vi "Format table.vi"(11 "Table输入":refnum<vi>) -> ()   [LabVIEW 2016]
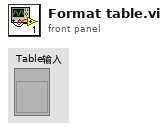
[diagram p1: front panel]
types:
  T1 = cluster{"Font Name:":string, "Size":i16, "Strikeout?":bool, "Italic?":bool, "Underline?":bool, "Outline?":bool, "Shadow?":bool, "Bold?":bool}
  T2 = enum16{"User-specified Font", "Application Font", "System Font", "Dialog Font"}
  T3 = typedef "LVFontTypeDef.ctl" = cluster{"Font Name":string, "Size":u16, "Bold":bool, "Italic":bool, "Underline":bool, "Strikeout":bool, "Color":u32}
  T4 = cluster{"left":i16, "top":i16, "right":i16, "bottom":i16}
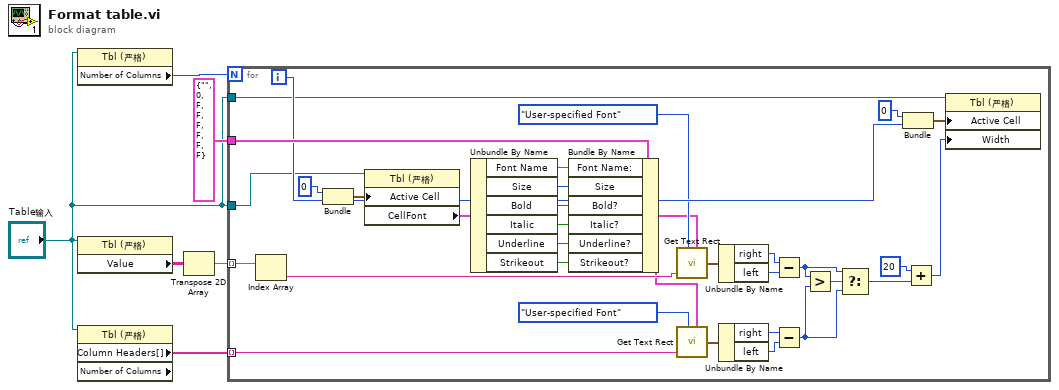
[diagram p0: block diagram]
diagram:
  n1 = property on="属性节点" class="Tbl (严格)"(reference="Table输入") -> ("Number of Columns"=w5:u32)  [unwired: 1 in, 2 out]
  n2 = property class="Tbl (严格)"(reference="Table输入") -> ("Value"=w6:string[][])  [unwired: 1 in, 2 out]
  n3 = property class="Tbl (严格)" props=["Column Headers[]", "Number of Columns"](reference="Table输入") -> ("Column Headers[]"=w1:string[])  [unwired: 1 in, 3 out]
  n4 = Transpose 2D Array(2D array=w6) -> (transposed array=w4:string[][])
  n5 = for {
    N: w5 -> [_]
    tunnel: w4 -> [w19] mode=indexing
    tunnel: T1 {"Font Name:"="", "Size"=0, "Strikeout?"=FALSE, "Italic?"=FALSE, "Underline?"=FALSE, "Outline?"=FALSE, "Shadow?"=FALSE, "Bold?"=FALSE} ("[user-specified font]") -> [w39]
    tunnel: "Table输入" -> [w33]
    tunnel: "Table输入" -> [w32]
    tunnel: w1 -> [w14] mode=indexing
    i -> [w38]
    n6 = Index Array(array=w19) -> (element=w18:string)  [unwired: 1 in]
    n7 = Bundle(0, w38) -> (w20:cluster{i32, i32})  [unwired: 1 in]
    n8 = property on="属性节点" class="Tbl (严格)"(reference=w33, "Active Cell"=w20) -> ("CellFont"=w21:T3)  [unwired: 1 in, 2 out]
    n9 = Unbundle By Name(w21) -> ("Font Name"=w31:string, "Size"=w30:u16, "Bold"=w29:bool, "Italic"=w28:bool, "Underline"=w27:bool, "Strikeout"=w26:bool)
    n10 = Bundle By Name(cluster=w39, "Font Name:"=w31, "Size"=w30, "Bold?"=w29, "Italic?"=w28, "Underline?"=w27, "Strikeout?"=w26) -> (w16:T1)
    n11 = call <vilib>:"Get Text Rect.vi"("desired font(Application)"=T2."User-specified Font", "text"=w18, "[user-specified font]"=w16) -> ("rect"=w24:T4)  [unwired: 6 in]
    n12 = call <vilib>:"Get Text Rect.vi"("desired font(Application)"=T2."User-specified Font", "text"=w14, "[user-specified font]"=w16) -> ("rect"=w11:T4)  [unwired: 6 in]
    n13 = Unbundle By Name(w24) -> ("right"=w23:i16, "left"=w22:i16)
    n14 = Unbundle By Name(w11) -> ("right"=w12:i16, "left"=w13:i16)
    n15 = Subtract(x=w23, y=w22) -> (x-y=w9:i16)
    n16 = Subtract(x=w12, y=w13) -> (x-y=w8:i16)
    n17 = Greater?(x=w9, y=w8) -> (0:w10:bool)
    n18 = Select(t=w9, s=w10, f=w8) -> (s? t:f=w7:i16)
    n19 = Bundle(0, w38) -> (w34:cluster{i32, i32})  [unwired: 1 in]
    n20 = Add(x=i16 20, y=w7) -> (x+y=w35:i16)
    n21 = property on="属性节点" class="Tbl (严格)"(reference=w32, "Active Cell"=w34, "Width"=w35) -> ()  [unwired: 1 in, 2 out]
  }
